vi "Upload_To_ADAM_Server.vi"(1 "First Loop":bool, 2 "Averaging Period (s)":dbl=1.0, 3 "Shift In":dbl[](array[numeric]), 4 "Channel Values":dbl[](array[numeric]), 5 "Give Variance":bool, 6 "Channel Names":string[](array[string])) -> (0 "Shift Out":dbl[](array[numeric]))   [LabVIEW 2011]
uses:
  ADAM Controls/Update_scan_value.ctl
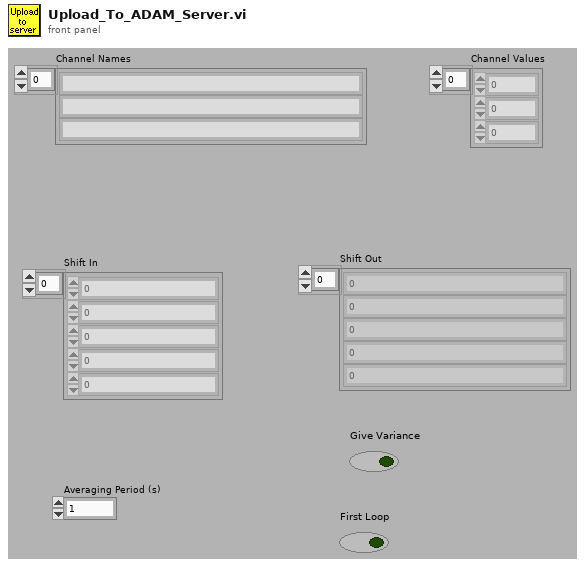
[diagram p1: front panel]
types:
  T1 = typedef "Update_scan_value.ctl" = cluster{"Channel Name":string, "New Value":dbl}
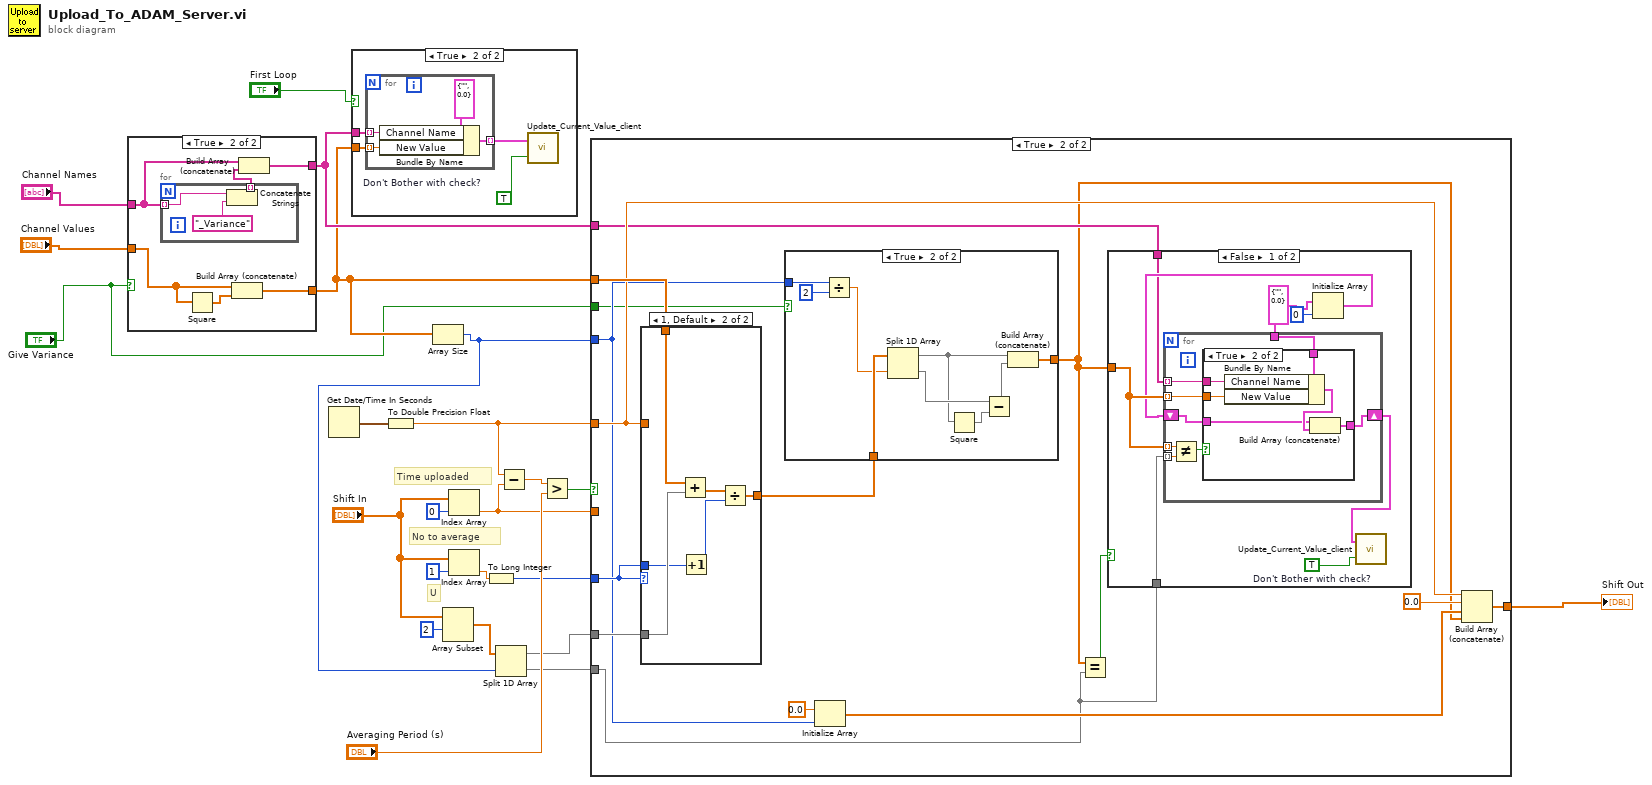
[diagram p0: block diagram]
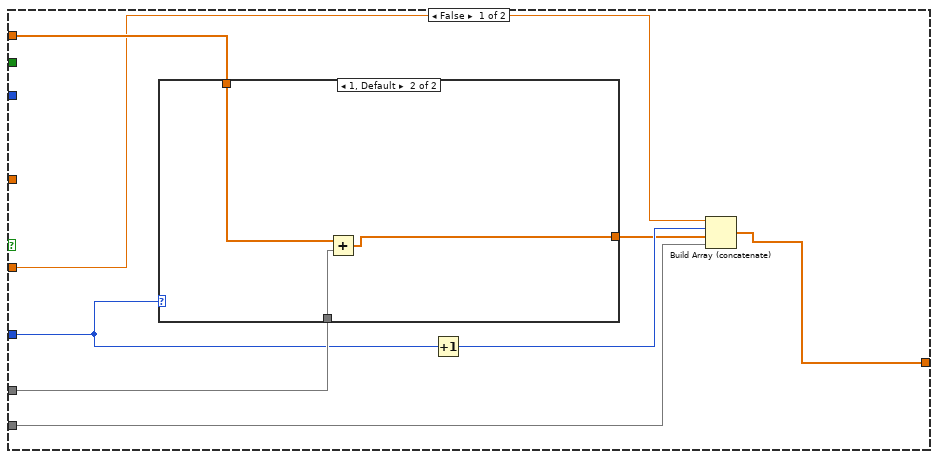
[diagram p4: hidden frame]
diagram:
  # "U"
  # "No to average"
  # "Time uploaded"
  n1 = case shown="True" "Give Variance" {
    tunnel: "Channel Names" -> [w25 w31]
    tunnel: [w25 w29] -> w4
    tunnel: "Channel Values" -> [w24 w27]
    tunnel: [w24 w26] -> w2
    frame False {
    }
    frame True {
      n2 = for {
        tunnel: w31 -> [w33] mode=indexing
        tunnel: [w32] -> w30 mode=indexing
        n3 = Concatenate Strings(w33, "_Variance") -> (w32:string)
      }
      n4 = Square(x=w27) -> (x^2=w28:dbl[])
      n5 = Build Array (concatenate)(w27, w28) -> (w26:dbl[])
      n6 = Build Array (concatenate)(w31, w30) -> (w29:string[])
    }
  }
  n7 = Get Date/Time In Seconds() -> (seconds since 1Jan1904=w22:timestamp)
  n8 = case shown="True" "First Loop" {
    tunnel: w4 -> [_ w36]
    tunnel: w2 -> [_ w35]
    frame False {
    }
    frame True {
      w38 = TRUE  # Don't Bother with check?
      n9 = for {
        tunnel: [w41] -> w37 mode=indexing
        tunnel: w36 -> [w40] mode=indexing
        tunnel: w35 -> [w39] mode=indexing
        n10 = Bundle By Name(cluster=T1 {"Channel Name"="", "New Value"=0.0} ("Update Scan Value Cluster"), "Channel Name"=w40, "New Value"=w39) -> (w41:T1)
      }
      n11 = call "Update_Current_Value_client.vi"("Don't Bother with check?"=w38, "Update array in"=w37) -> ()
    }
  }
  n12 = To Double Precision Float(number=w22) -> (double precision float=w13:dbl)
  n13 = Array Size(array=w2) -> (size(s)=w9:i32)
  n14 = Array Subset(array="Shift In", index=2) -> (w10:dbl[])  [unwired: 1 in]
  n15 = Index Array(array="Shift In", index=0) -> (element=w11:dbl)
  n16 = Index Array(array="Shift In", index=1) -> (element=w15:dbl)
  n17 = To Long Integer(number=w15) -> (32bit integer=w14:i32)
  n18 = Split 1D Array(array=w10, index=w9) -> (first subarray=w8:dbl[], second subarray=w7:dbl[])
  n19 = Subtract(x=w13, y=w11) -> (x-y=w21:dbl)
  n20 = Greater?(x=w21, y="Averaging Period (s)") -> (0:w19:bool)
  n21 = case shown="True" w19 {
    tunnel: w2 -> [w50 w69]
    tunnel: w8 -> [w49 w64]
    tunnel: w14 -> [w47 w68]
    tunnel: w13 -> [_ w67]
    tunnel: [w44 w65] -> w12
    tunnel: w11 -> [w48 _]
    tunnel: w9 -> [_ w58]
    tunnel: w7 -> [w43 w60]
    tunnel: w4 -> [_ w59]
    tunnel: "Give Variance" -> [_ w55]
    frame False {
      n22 = case shown="1, Default" w47 {
        tunnel: w50 -> [w51 w54]
        tunnel: w49 -> [_ w53]
        tunnel: [w51 w52] -> w45
        frame 0 {
        }
        frame 1, Default {
          n23 = Add(x=w54, y=w53) -> (x+y=w52:dbl[])
        }
      }
      n24 = Increment(x=w47) -> (x+1=w46:i32)
      n25 = Build Array (concatenate)(w48, w46, w45, w43) -> (w44:dbl[])
    }
    frame True {
      n26 = case shown="1, Default" w68 {
        tunnel: w67 -> [_ _]
        tunnel: w64 -> [_ w108]
        tunnel: w69 -> [w103 w109]
        tunnel: w68 -> [_ w107]
        tunnel: [w103 w104] -> w57
        frame 0 {
        }
        frame 1, Default {
          n27 = Add(x=w109, y=w108) -> (x+y=w106:dbl[])
          n28 = Increment(x=w107) -> (x+1=w105:i32)
          n29 = Divide(x=w106, y=w105) -> (x/y=w104:dbl[])
        }
      }
      n30 = case shown="True" w55 {
        tunnel: w58 -> [_ w79]
        tunnel: w57 -> [w70 w77]
        tunnel: [w70 w72] -> w56
        frame False {
        }
        frame True {
          n31 = Divide(x=w79, y=2) -> (x/y=w76:dbl)
          n32 = Split 1D Array(array=w77, index=w76) -> (first subarray=w74:dbl[], second subarray=w75:dbl[])
          n33 = Square(x=w74) -> (x^2=w71:dbl[])
          n34 = Subtract(x=w75, y=w71) -> (x-y=w73:dbl[])
          n35 = Build Array (concatenate)(w74, w73) -> (w72:dbl[])
        }
      }
      n36 = Initialize Array(0.0 ("element"), w58) -> (w62:dbl[])
      n37 = Equal?(x=w56, y=w60) -> (x = y?=w61:bool)
      n38 = case shown="False" w61 {
        tunnel: w56 -> [w86 _]
        tunnel: w60 -> [w85 _]
        tunnel: w59 -> [w80 _]
        frame False {
          w87 = TRUE  # Don't Bother with check?
          w84 = T1 {"Channel Name"="", "New Value"=0.0} ("Update Scan Value Cluster")
          n39 = Initialize Array(w84, 0 ("dimension size")) -> (w82:T1[])
          n40 = for {
            tunnel: w84 -> [w95]
            tunnel: w80 -> [w94] mode=indexing
            tunnel: w86 -> [w93] mode=indexing
            shift-right: [w89] -> w81
            shift-left: w82 -> [w90]
            tunnel: w86 -> [w92] mode=indexing
            tunnel: w85 -> [w91] mode=indexing
            n41 = Not Equal?(x=w92, y=w91) -> (x != y?=w88:bool)
            n42 = case shown="True" w88 {
              tunnel: w95 -> [_ w102]
              tunnel: w94 -> [_ w101]
              tunnel: w93 -> [_ w100]
              tunnel: w90 -> [w96 w98]
              tunnel: [w96 w97] -> w89
              frame False {
              }
              frame True {
                n43 = Bundle By Name(cluster=w102, "Channel Name"=w101, "New Value"=w100) -> (w99:T1)
                n44 = Build Array (concatenate)(w98, w99) -> (w97:T1[])
              }
            }
          }
          n45 = call "Update_Current_Value_client.vi"("Don't Bother with check?"=w87, "Update array in"=w81) -> ()
        }
        frame True {
        }
      }
      n46 = Build Array (concatenate)(w67, 0.0 ("element"), w62, w56) -> (w65:dbl[])
    }
  }
  "Shift Out" <- w12
